vi "Init.vi"(8 "error in":errorcluster, 11 "XNET Base CFG in":refnum<class "XNET Base CFG.lvclass">) -> (0 "error out":errorcluster, 3 "XNET Base CFG out":refnum<class "XNET Base CFG.lvclass">)   [LabVIEW 2024, in "XNET Base CFG.lvclass"]
uses:
  XNET Base CFG.lvclass
  Configurations/CFG Base/CFG Base.lvclass
  XNET Base CFG.lvclass/XNET Base CFG.ctl
  D:/git/HAL/HAL/Configurations/CFG Base/CFG Base.lvclass
  D:/git/HAL/HAL/Devices/CAN Interfaces/XNET/XNET Base CFG/XNET Base CFG.lvclass
  D:/git/HAL/HAL/Protocols/ICAN/ICAN.lvclass
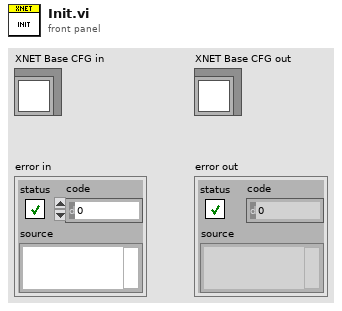
[diagram p1: front panel]
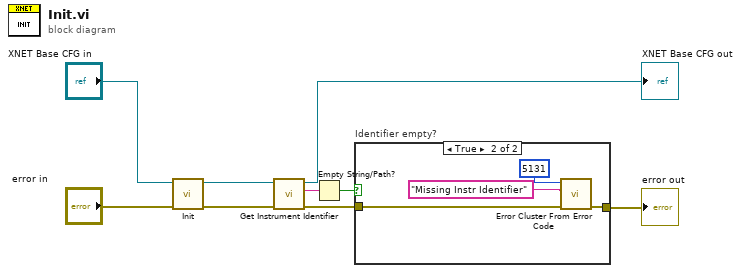
[diagram p0: block diagram]
diagram:
  n1 = call-parent "Init.vi"("error in"="error in", "CFG Base in"="XNET Base CFG in") -> ("error out"=w1:errorcluster, "CFG Base out"=w2:refnum<class "XNET Base CFG.lvclass">)  [unwired: 8 in]
  n2 = call "Get Instrument Identifier.vi"("CFG Base in"=w2) -> ("Instrument Identifier"=w7:string, "CFG Base out"=→"XNET Base CFG out":refnum<class "XNET Base CFG.lvclass">)  [unwired: 9 in]
  n3 = Empty String/Path?(string/path=w7) -> (empty?=w8:bool)
  n4 = case "Identifier empty?" shown="True" w8 {
    tunnel: w1 -> [w9 w13]
    tunnel: [w9 w12] -> w4
    frame False {
    }
    frame True {
      n5 = call <vilib>:"Error Cluster From Error Code.vi"("error in (no error)"=w13, "error message (\"\")"="Missing Instr Identifier" ("error message (\"\")"), "error code (0)"=5131) -> ("error out"=w12:errorcluster)  [unwired: 6 in]
    }
  }
  "error out" <- w4
